vi "Andor_Cam.vi"(0 "Operation":T2(ring), 1 "Camera-specific in":variant, 5 "Exposure time (s)":dbl, 7 "Save path":path, 9 "Capture mode":enum16{"Single frame", "Sequence"}(ring), 11 "Capture button":refnum<vi>, 12 "Image in":variant, 14 "Frames in sequence":u32) -> (3 "Camera-specific out":variant, 4 "Status":T1)   [LabVIEW 2018]
uses:
  <userlib>/atmcd32d.llb/AcquisitionMode_mode typedef.ctl
  <userlib>/atmcd32d.llb/ReadMode_mode typedef.ctl
  <userlib>/atmcd32d.llb/HSSpeed_type typedef.ctl
  <userlib>/atmcd32d.llb/TriggerMode_mode typedef.ctl
  <userlib>/atmcd32d.llb/Shutter_type typedef.ctl
  <userlib>/atmcd32d.llb/Shutter_mode typedef.ctl
  <vilib>/vision/Image Controls.llb/IMAQ Image.ctl
  <userlib>/atmcd32d.llb/Error Code Enum typedef.ctl
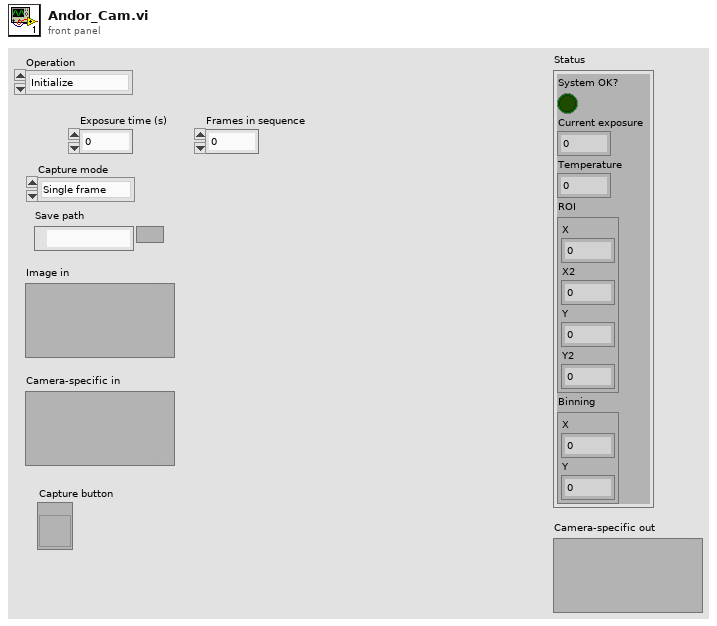
[diagram p1: front panel]
types:
  T1 = cluster{"System OK?":bool, "Current exposure":dbl, "Temperature":dbl, "ROI":cluster{"X":u32, "X2":u32, "Y":u32, "Y2":u32}, "Binning":cluster{"X":u32, "Y":u32}}
  T2 = enum16{"Initialize", "Shut down", "Set capture mode", "Set exposure", "Trigger and read", "Get status", "Other settings"}
  T3 = typedef "ReadMode_mode typedef.ctl" = enum16{"Full Vertical Binning", "Multi-Track", "Random-Track", "Single-Track", "Image"}
  T4 = typedef "HSSpeed_type typedef.ctl" = enum16{"EM Amp", "Conventional Amp"}
  T5 = typedef "TriggerMode_mode typedef.ctl" = enum16{"Internal", "External", "N/A (2)", "N/A (3)", "N/A (4)", "N/A (5)", "External Start", "External Exposure (Bulb)", "N/A (8)", "External FVB EM", "Software", "N/A (11)", "External Charge Shifting"}
  T6 = typedef "Shutter_mode typedef.ctl" = enum16{"Auto", "Open", "Close", "N/A (3)", "Open FVB Series", "Open Any Series"}
  T7 = typedef "AcquisitionMode_mode typedef.ctl" = enum16{"Reserved (0)", "Single Scan", "Accumulate", "Kinetics", "Fast Kinetics", "Run Till Abort", "Reserved (6)", "Reserved (7)", "Reserved (8)", "Time Delayed Integration"}
  T8 = typedef "IMAQ Image.ctl" = refnum<image>
  T9 = cluster{"New Image":T8, "Image":refnum<vi>, "FPS target":dbl}
  T10 = typedef "Error Code Enum typedef.ctl" = enum32{"N/A (0)", "DRV_ERROR_CODES", "DRV_SUCCESS", "DRV_VXDNOTINSTALLED", "DRV_ERROR_SCAN", "DRV_ERROR_CHECK_SUM", "DRV_ERROR_FILELOAD", "DRV_UNKNOWN_FUNC", "DRV_ERROR_VXD_INIT", "DRV_ERROR_ADDRESS", "DRV_ERROR_PAGELOCK", "DRV_ERROR_PAGEUNLOCK", "DRV_ERROR_BOARDTEST", "DRV_ERROR_ACK", "DRV_ERROR_UP_FIFO", "DRV_ERROR_PATTERN", "N/A (16)", "DRV_ACQUISITION_ERRORS", "DRV_ACQ_BUFFER", "DRV_ACQ_DOWNFIFO_FULL", "DRV_PROC_UNKONWN_INSTRUCTION", "DRV_ILLEGAL_OP_CODE", "DRV_KINETIC_TIME_NOT_MET", "DRV_ACCUM_TIME_NOT_MET", "DRV_NO_NEW_DATA", "N/A (25)", "DRV_SPOOLERROR", "N/A (27)", "N/A (28)", "N/A (29)", "N/A (30)", "N/A (31)", "N/A (32)", "DRV_TEMPERATURE_CODES", "DRV_TEMPERATURE_OFF", "DRV_TEMPERATURE_NOT_STABILIZED", "DRV_TEMPERATURE_STABILIZED", "DRV_TEMPERATURE_NOT_REACHED", "DRV_TEMPERATURE_OUT_RANGE", "DRV_TEMPERATURE_NOT_SUPPORTED", "DRV_TEMPERATURE_DRIFT", "N/A (41)", "N/A (42)", "N/A (43)", "N/A (44)", "N/A (45)", "N/A (46)", "N/A (47)", "N/A (48)", "DRV_GENERAL_ERRORS", "DRV_INVALID_AUX", "DRV_COF_NOTLOADED", "DRV_FPGAPROG", "DRV_FLEXERROR", "DRV_GPIBERROR", "N/A (55)", "N/A (56)", "N/A (57)", "N/A (58)", "N/A (59)", "N/A (60)", "N/A (61)", "N/A (62)", "N/A (63)", "DRV_DATATYPE", "DRV_DRIVER_ERRORS", "DRV_P1INVALID", "DRV_P2INVALID", "DRV_P3INVALID", "DRV_P4INVALID", "DRV_INIERROR", "DRV_COFERROR", "DRV_ACQUIRING", "DRV_IDLE", "DRV_TEMPCYCLE", "DRV_NOT_INITIALIZED", "DRV_P5INVALID", "DRV_P6INVALID", "DRV_INVALID_MODE", "DRV_INVALID_FILTER", "DRV_I2CERRORS", "DRV_I2CDEVNOTFOUND", "DRV_I2CTIMEOUT", "DRV_P7INVALID", "N/A (84)", "N/A (85)", "N/A (86)", "N/A (87)", "N/A (88)", "N/A (89)", "DRV_IOCERROR", "DRV_VRMVERSIONERROR"}
  T11 = enum16{"open", "replace", "create", "open or create", "replace or create", "replace or create with confirmation"}
  T12 = typedef "Shutter_type typedef.ctl" = enum16{"TTL Low", "TTL High"}
  T13 = cluster{"File refnum":refnum<file>, "Image File Directory":cluster{cluster{"Field":u16, "Type":u16, "Count":u32, "Value / Offset":u32, "Add IFD Offset?":bool}[], cluster{"Data":u32[], "Add offset?":bool}[]}, "Big endian?":bool, "IFD Offset Size":u32}
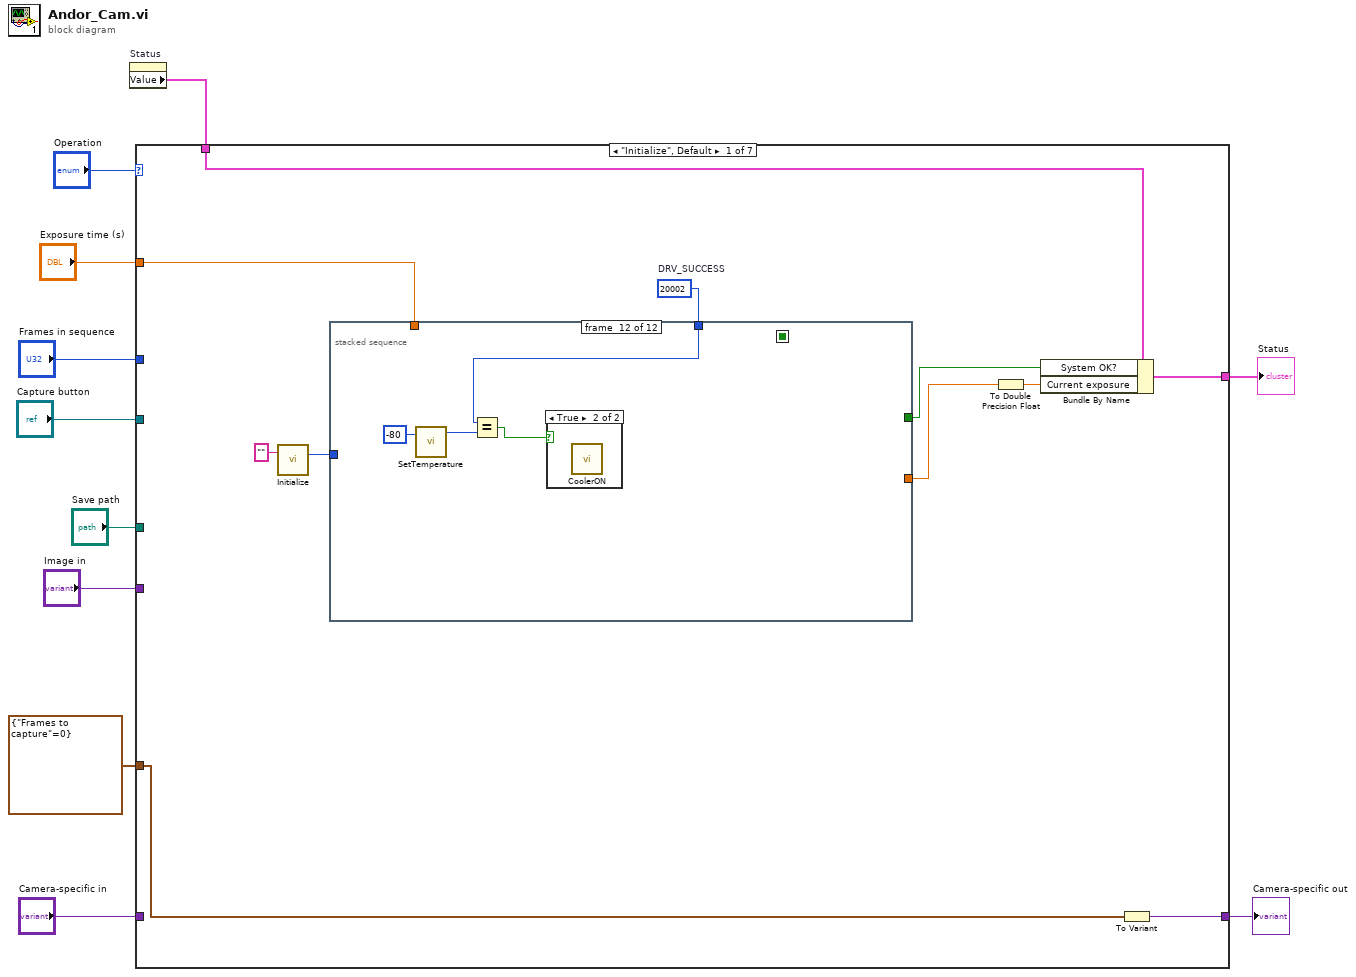
[diagram p0: block diagram]
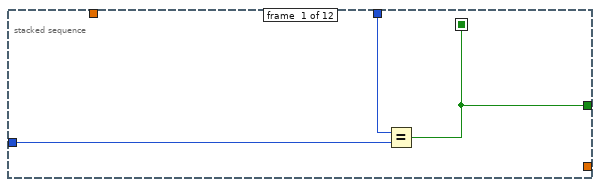
[diagram p2: hidden frame]
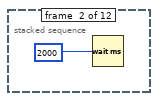
[diagram p3: hidden frame]
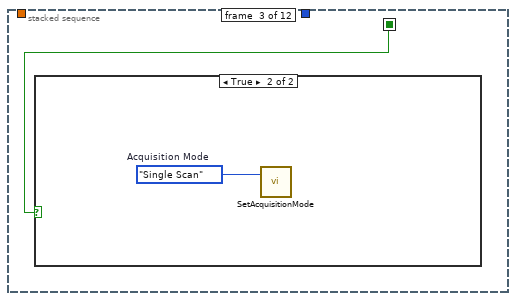
[diagram p4: hidden frame]
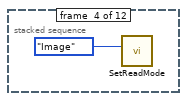
[diagram p6: hidden frame]
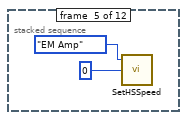
[diagram p7: hidden frame]
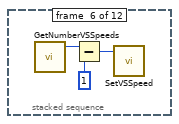
[diagram p8: hidden frame]
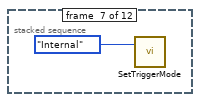
[diagram p9: hidden frame]
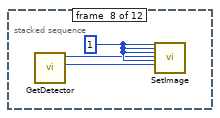
[diagram p10: hidden frame]
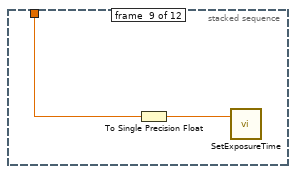
[diagram p11: hidden frame]
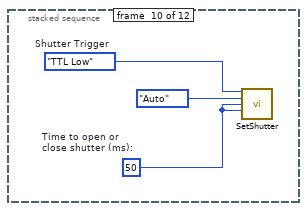
[diagram p12: hidden frame]
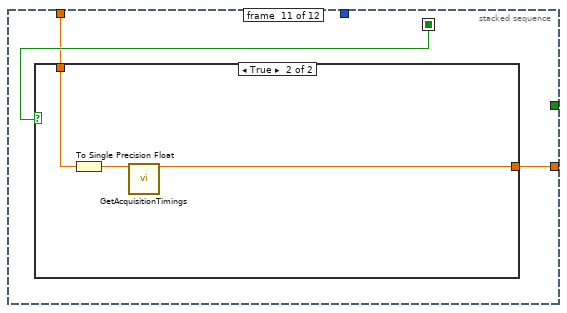
[diagram p13: hidden frame]
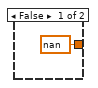
[diagram p14: hidden frame]
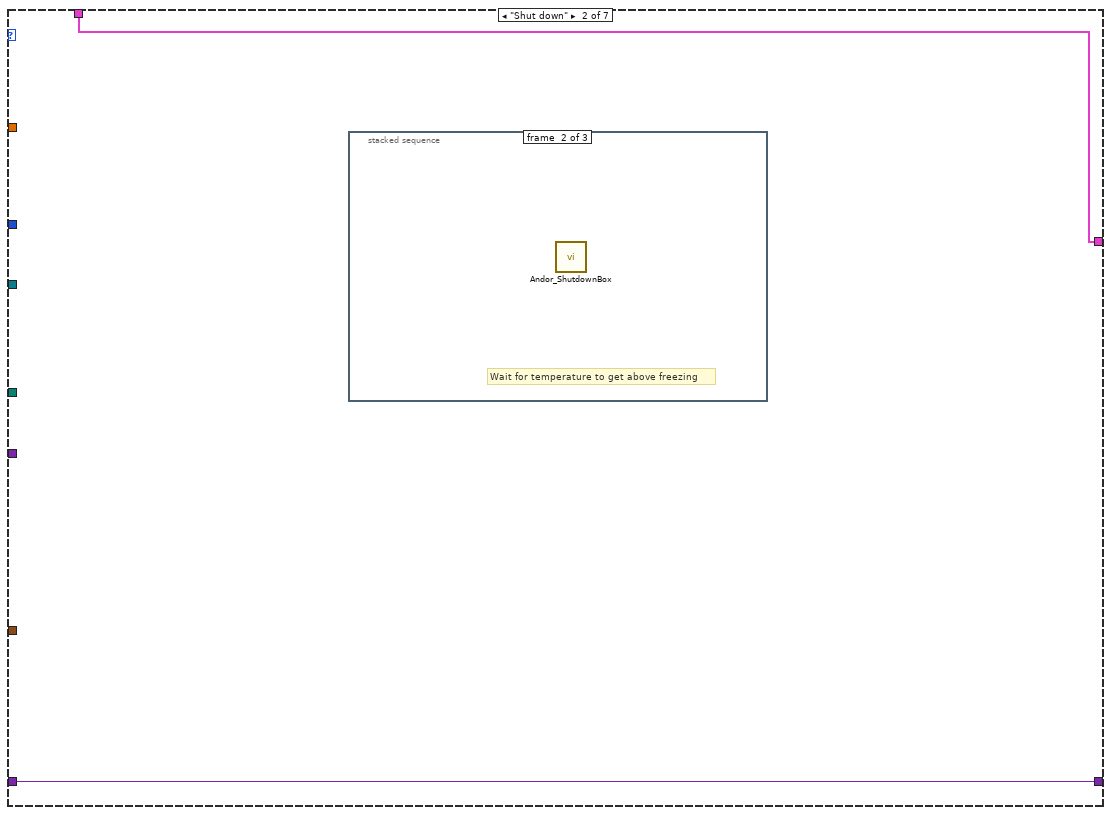
[diagram p16: hidden frame]
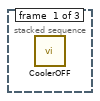
[diagram p17: hidden frame]
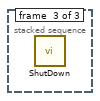
[diagram p18: hidden frame]
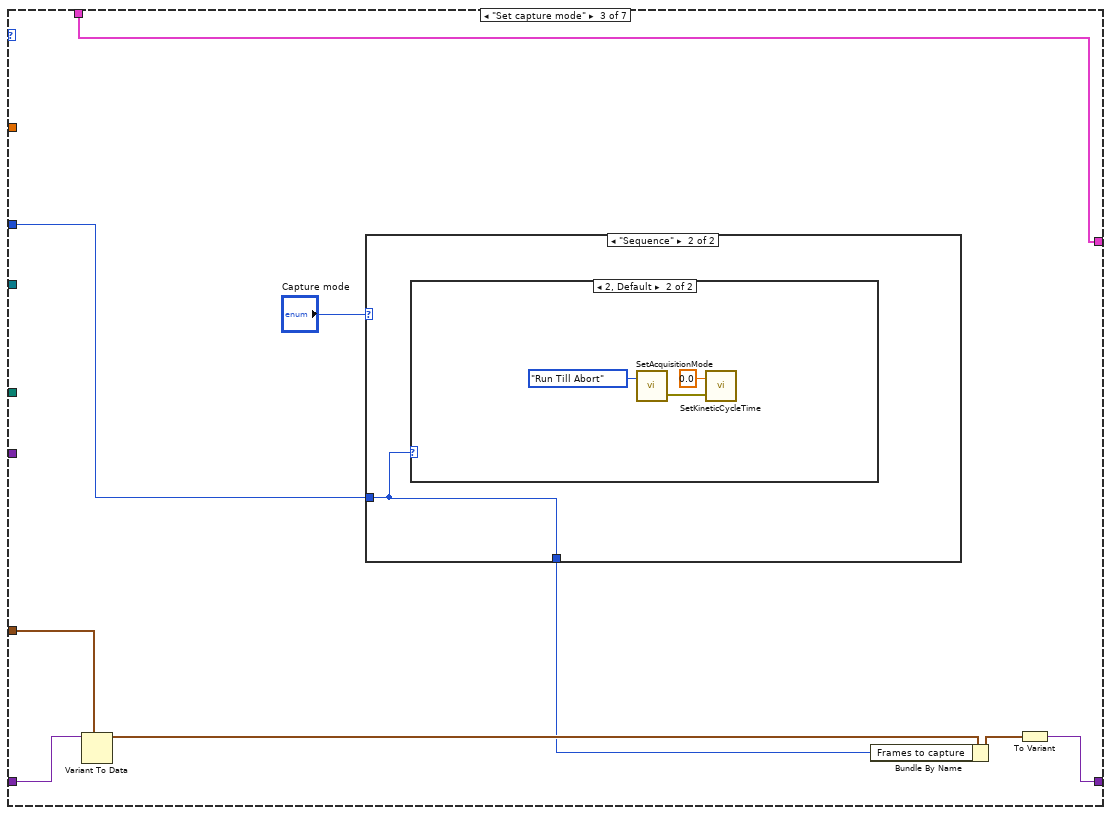
[diagram p19: hidden frame]
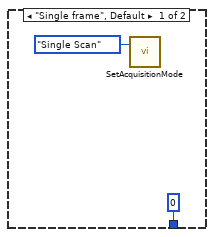
[diagram p20: hidden frame]
diagram:
  n1 = property on="Status" class="Clust (strict)"() -> ("Value"=w9:T1)  [unwired: 2 in, 2 out]
  n2 = case shown="\"Initialize\", Default" "Operation" {
    tunnel: "Exposure time (s)" -> [w19 _ _ w76 _ _ _]
    tunnel: w9 -> [w18 w56 w65 w78 w93 w321 w323]
    tunnel: [w17 w56 w65 w75 w93 w320 w323] -> w8
    tunnel: "Save path" -> [_ _ _ _ w92 _ _]
    tunnel: "Image in" -> [_ _ _ _ w85 _ _]
    tunnel: [w13 w55 w60 w73 w91 w316 w322] -> w5
    tunnel: "Camera-specific in" -> [_ w55 w63 w73 w91 w316 w322]
    tunnel: cluster{"Frames to capture":u32} {"Frames to capture"=0} -> [w14 _ w62 _ w90 _ _]
    tunnel: "Frames in sequence" -> [_ _ w57 _ _ _ _]
    tunnel: "Capture button" -> [_ _ _ _ w83 _ _]
    frame "Initialize", Default {
      w20 = u32 20002  # DRV_SUCCESS
      n3 = call <userlib>:"Initialize.vi"("directory (\"\")"="" ("directory (\"\")")) -> ("DLL error code"=w21:u32)  [unwired: 1 in, 1 out]
      n4 = stacked-sequence {
        seq-local: [w23 _ _ _ _ _ _ _ _ _ _ _] -> [_ _ w27 _ _ _ _ _ _ _ w46 _]
        tunnel: w19 -> [_ _ _ _ _ _ _ _ w40 _ w45 _]
        tunnel: w20 -> [w25 _ _ _ _ _ _ _ _ _ _ w52]
        tunnel: w21 -> [w24 _ _ _ _ _ _ _ _ _ _ _]
        tunnel: [w23 _ _ _ _ _ _ _ _ _ _ _] -> w16
        tunnel: [_ _ _ _ _ _ _ _ _ _ w44 _] -> w15
        frame #0 {
          n5 = Equal?(x=w25, y=w24) -> (x = y?=w23:bool)
        }
        frame #1 {
          n6 = Wait (ms)(milliseconds to wait=u32 2000) -> ()  [unwired: 1 out]
        }
        frame #2 {
          n7 = case shown="True" w27 {
            frame False {
            }
            frame True {
              w28 = AcquisitionMode_mode_typedef."Single Scan"  # Acquisition Mode
              n8 = call <userlib>:"SetAcquisitionMode.vi"("mode"=w28) -> ()  [unwired: 1 in, 2 out]
            }
          }
        }
        frame #3 {
          n9 = call <userlib>:"SetReadMode.vi"("mode"=ReadMode_mode_typedef."Image") -> ()  [unwired: 1 in, 2 out]
        }
        frame #4 {
          n10 = call <userlib>:"SetHSSpeed.vi"("index"=0, "type"=HSSpeed_type_typedef."EM Amp") -> ()  [unwired: 2 in, 2 out]
        }
        frame #5 {
          n11 = call <userlib>:"GetNumberVSSpeeds.vi"() -> ("number"=w34:i32)  [unwired: 3 in, 2 out]
          n12 = Subtract(x=w34, y=1) -> (x-y=w32:i32)
          n13 = call <userlib>:"SetVSSpeed.vi"("index"=w32) -> ()  [unwired: 1 in, 2 out]
        }
        frame #6 {
          n14 = call <userlib>:"SetTriggerMode.vi"("mode"=TriggerMode_mode_typedef."Internal") -> ()  [unwired: 1 in, 2 out]
        }
        frame #7 {
          w38 = 1 ("hbin")
          n15 = call <userlib>:"GetDetector.vi"() -> ("ypixels"=w36:i32, "xpixels"=w37:i32)  [unwired: 4 in, 2 out]
          n16 = call <userlib>:"SetImage.vi"("hbin"=w38, "vbin"=w38, "hstart"=w38, "hend"=w37, "vstart"=w38, "vend"=w36) -> ()  [unwired: 20 in, 2 out]
        }
        frame #8 {
          n17 = To Single Precision Float(number=w40) -> (single precision float=w39:sgl)
          n18 = call <userlib>:"SetExposureTime.vi"("time"=w39) -> ()  [unwired: 1 in, 2 out]
        }
        frame #9 {
          w43 = 50  # Time to open or close shutter (ms):
          w42 = Shutter_type_typedef."TTL Low"  # Shutter Trigger
          n19 = call <userlib>:"SetShutter.vi"("type"=w42, "mode"=Shutter_mode_typedef."Auto", "closingtime"=w43, "openingtime"=w43) -> ()  [unwired: 10 in, 2 out]
        }
        frame #10 {
          n20 = case shown="True" w46 {
            tunnel: w45 -> [_ w50]
            tunnel: [sgl nan ("exposure") w49] -> w44
            frame False {
            }
            frame True {
              n21 = To Single Precision Float(number=w50) -> (single precision float=w48:sgl)
              n22 = call <userlib>:"GetAcquisitionTimings.vi"("exposure input"=w48) -> ("exposure"=w49:sgl)  [unwired: 10 in, 4 out]
            }
          }
        }
        frame #11 {
          n23 = call <userlib>:"SetTemperature.vi"("temperature"=-80) -> ("DLL error code"=w53:u32)  [unwired: 1 in, 1 out]
          n24 = Equal?(x=w52, y=w53) -> (x = y?=w51:bool)
          n25 = case shown="True" w51 {
            frame False {
            }
            frame True {
              n26 = call <userlib>:"CoolerON.vi"() -> ()  [unwired: 2 in, 2 out]
            }
          }
        }
      }
      n27 = To Double Precision Float(number=w15) -> (double precision float=w12:dbl)
      n28 = Bundle By Name(cluster=w18, "System OK?"=w16, "Current exposure"=w12) -> (w17:T1)
      n29 = To Variant(anything=w14) -> (Variant=w13:variant)
    }
    frame "Shut down" {
      n30 = stacked-sequence {
        frame #0 {
          n31 = call <userlib>:"CoolerOFF.vi"() -> ()  [unwired: 2 in, 2 out]
        }
        frame #1 {
          # "Wait for temperature to get above freezing"
          n32 = call "Andor_ShutdownBox.vi"() -> ()  [unwired: 12 in]
        }
        frame #2 {
          n33 = call <userlib>:"ShutDown.vi"() -> ()  [unwired: 2 in, 2 out]
        }
      }
    }
    frame "Set capture mode" {
      n34 = Variant To Data(type=w62, Variant=w63) -> (data=w61:cluster{"Frames to capture":u32})  [unwired: 1 in, 1 out]
      n35 = case shown="\"Sequence\"" "Capture mode" {
        tunnel: [u32 0 ("Frames in sequence") w68] -> w58
        tunnel: w57 -> [_ w68]
        frame "Single frame", Default {
          n36 = call <userlib>:"SetAcquisitionMode.vi"("mode"=AcquisitionMode_mode_typedef."Single Scan") -> ()  [unwired: 1 in, 2 out]
        }
        frame "Sequence" {
          n37 = case shown="2, Default" w68 {
            frame 0, 1 {
              n38 = call <userlib>:"SetAcquisitionMode.vi"("mode"=AcquisitionMode_mode_typedef."Single Scan") -> ()  [unwired: 1 in, 2 out]
            }
            frame 2, Default {
              n39 = call <userlib>:"SetAcquisitionMode.vi"("mode"=AcquisitionMode_mode_typedef."Run Till Abort") -> ("error out"=w70:errorcluster)  [unwired: 1 in, 1 out]
              n40 = call <userlib>:"SetKineticCycleTime.vi"("error in (no error)"=w70, "time"=sgl 0.0) -> ()  [unwired: 2 out]
            }
          }
        }
      }
      n41 = Bundle By Name(cluster=w61, "Frames to capture"=w58) -> (w59:cluster{"Frames to capture":u32})
      n42 = To Variant(anything=w59) -> (Variant=w60:variant)
    }
    frame "Set exposure" {
      n43 = To Single Precision Float(number=w76) -> (single precision float=w77:sgl)
      n44 = stacked-sequence {
        tunnel: w77 -> [w79 w81]
        tunnel: [_ w80] -> w74
        frame #0 {
          n45 = call <userlib>:"SetExposureTime.vi"("time"=w79) -> ()  [unwired: 1 in, 2 out]
        }
        frame #1 {
          n46 = call <userlib>:"GetAcquisitionTimings.vi"("exposure input"=w81) -> ("exposure"=w80:sgl)  [unwired: 10 in, 4 out]
        }
      }
      n47 = Bundle By Name(cluster=w78, "Current exposure"=w74) -> (w75:T1)
    }
    frame "Trigger and read" {
      n48 = Variant To Data(type=w90, Variant=w91) -> (data=w89:cluster{"Frames to capture":u32})  [unwired: 1 in, 1 out]
      n49 = Unbundle By Name(w89) -> ("Frames to capture"=w88:u32)
      n50 = Variant To Data(type=T9 {"New Image"=refnum, "Image"=refnum, "FPS target"=0.0} ("output cluster"), Variant=w85) -> (data=w87:T9)  [unwired: 1 in, 1 out]
      n51 = Unbundle(w87) -> ("New Image"=w84:T8, "Image"=w82:refnum<vi>)  [unwired: 1 out]
      n52 = case shown="2, Default" w88 {
        selector: w88 -> [_ w151]
        tunnel: w92 -> [w96 w154]
        tunnel: w84 -> [w95 w153]
        tunnel: w83 -> [_ w152]
        tunnel: w82 -> [w94 w150]
        frame 0, 1 {
          n53 = stacked-sequence {
            seq-local: [w99 _ _] -> [_ w100 _]
            tunnel: w96 -> [_ _ w112]
            tunnel: w95 -> [_ _ w110]
            tunnel: w94 -> [_ _ w105]
            frame #0 {
              w97 = u32 20002  # DRV_SUCCESS
              n54 = call <userlib>:"StartAcquisition.vi"() -> ("DLL error code"=w98:u32)  [unwired: 2 in, 1 out]
              n55 = Equal?(x=w97, y=w98) -> (x = y?=w99:bool)
            }
            frame #1 {
              n56 = case shown="True" w100 {
                frame False {
                }
                frame True {
                  n57 = while {
                    stop <- w103 continue-if-true
                    n58 = call <userlib>:"GetStatus.vi"() -> ("status"=w102:T10)  [unwired: 3 in, 2 out]
                    n59 = Wait Until Next ms Multiple(millisecond multiple=u32 25) -> ()  [unwired: 1 out]
                    n60 = Equal?(x=w102, y=Error_Code_Enum_typedef."DRV_ACQUIRING" ("status")) -> (x = y?=w103:bool)
                  }
                }
              }
            }
            frame #2 {
              n61 = call <userlib>:"GetDetector.vi"() -> ("ypixels"=w106:i32, "xpixels"=w107:i32)  [unwired: 4 in, 2 out]
              n62 = Multiply(x=w107, y=w106) -> (x*y=w118:i32)
              n63 = To Unsigned Long Integer(number=w118) -> (unsigned 32bit integer=w114:u32)
              n64 = Not A Number/Path/Refnum?(number/path/refnum=w110) -> (NaN/Path/Refnum?=w109:bool)
              n65 = call <userlib>:"GetAcquiredData.vi"("size"=w114) -> ("array"=w116:i32[])  [unwired: 2 in, 2 out]
              n66 = Multiply(x=1, y=w116) -> (x*y=w115:i32[])
              n67 = Reshape Array(w115, w106, w107) -> (w111:i32[][])
              n68 = To Unsigned Word Integer(number=w111) -> (unsigned 16bit integer=w108:u16[][])
              n69 = case shown="False" w109 {
                tunnel: w110 -> [w122 _]
                tunnel: w108 -> [w121 _]
                tunnel: w105 -> [w120 _]
                frame False {
                  n70 = call "IMAQ ArrayToImage"("Image Pixels (U16)"=w121, "Image"=w122) -> ("Image Out"=w119:T8)  [unwired: 8 in, 1 out]
                  n71 = property class="ImageControl"(reference=w120, "Value"=w119) -> ()  [unwired: 1 in, 2 out]
                }
                frame True {
                }
              }
              n72 = Not A Number/Path/Refnum?(number/path/refnum=w112) -> (NaN/Path/Refnum?=w113:bool)
              n73 = case shown="False" w113 {
                tunnel: w112 -> [w126 _]
                tunnel: w108 -> [w127 _]
                tunnel: w107 -> [w124 _]
                tunnel: w106 -> [w123 _]
                frame False {
                  n74 = call <vilib>:"Get File Extension.vi"("file"=w126) -> ("lowercase file extension"=w125:string)  [unwired: 6 in, 4 out]
                  n75 = case shown="\"'tiff'\", \"tif\"" w125 {
                    tunnel: w126 -> [w142 w149]
                    tunnel: w127 -> [w132 w147]
                    tunnel: w124 -> [w140 _]
                    tunnel: w123 -> [w139 _]
                    frame "'tiff'", "tif" {
                      n76 = To Unsigned Long Integer(number=w139) -> (unsigned 32bit integer=w128:u32)
                      n77 = To Unsigned Long Integer(number=w140) -> (unsigned 32bit integer=w129:u32)
                      n78 = call "TIFFStream Open.vi"("Bytes per strip"=u32 8000, "File path"=w142, "Height Pixels"=w128, "Width Pixels"=w129, "Big endian?"=FALSE) -> ("error out"=w136:errorcluster, "Current and next IFD offset"=w134:u32[], "Image data reference"=w133:refnum<data-value>, "File data"=w138:T13)  [unwired: 3 in]
                      n79 = in-place {
                        in-place-border: w132 -> [w143]
                        n80 = in-place-dvr #1(w133) -> ()  [unwired: 2 out]
                        n81 = in-place-dvr #1(w143) -> (w131:refnum<data-value>)  [unwired: 1 out]
                      }
                      n82 = call "TIFFStream Write.vi"("File data"=w138, "error in (no error)"=w136, "Last image in file?"=TRUE, "Current and next IFD offset in"=w134, "Image data reference"=w131) -> ("error out"=w137:errorcluster)  [unwired: 4 in, 2 out]
                      n83 = call "TIFFStream Close.vi"("error in (no error)"=w137, "Image data reference"=w131, "File data"=w138) -> ()  [unwired: 8 in, 1 out]
                    }
                    frame "dat", Default {
                      n84 = Open/Create/Replace File(file path (use dialog)=w149, operation (0:open)=T11."replace or create") -> (refnum out=w148:refnum<file>)  [unwired: 4 in, 2 out]
                      n85 = Write to Binary File(file (use dialog)=w148, data=w147, 5:FALSE ("prepend array or string size? (T)")) -> (refnum out=w145:refnum<file>)  [unwired: 3 in, 2 out]
                      n86 = Close File(refnum=w145) -> ()  [unwired: 1 in, 2 out]
                    }
                  }
                }
                frame True {
                }
              }
            }
          }
        }
        frame 2, Default {
          n87 = stacked-sequence {
            seq-local: [_ w193 _ _ _] -> [_ _ _ _ _]
            seq-local: [w158 _ _ _ _] -> [_ _ w205 _ _]
            seq-local: [w166 _ _ _ _] -> [_ _ w207 _ w303]
            seq-local: [w162 _ _ _ _] -> [_ _ w204 _ _]
            seq-local: [w163 _ _ _ _] -> [_ _ w206 _ _]
            seq-local: [w161 _ _ _ _] -> [_ _ w203 _ _]
            seq-local: [w160 _ _ _ _] -> [_ _ w201 _ w300]
            seq-local: [w159 _ _ _ _] -> [_ _ w202 _ _]
            seq-local: [_ _ w200 _ _] -> [_ _ _ _ w299]
            seq-local: [_ _ w199 _ _] -> [_ _ _ _ w298]
            seq-local: [w156 _ _ _ _] -> [_ _ w198 _ _]
            seq-local: [w155 _ _ _ _] -> [_ _ w197 _ _]
            tunnel: w154 -> [w168 _ w210 _ w301]
            tunnel: w153 -> [_ _ w209 _ _]
            tunnel: w152 -> [_ _ w208 _ _]
            tunnel: w151 -> [_ _ w196 _ _]
            tunnel: w150 -> [_ _ w194 _ _]
            frame #0 {
              n88 = call <userlib>:"GetDetector.vi"() -> ("ypixels"=w162:i32, "xpixels"=w163:i32)  [unwired: 4 in, 2 out]
              n89 = To Unsigned Long Integer(number=w163) -> (unsigned 32bit integer=w165:u32)
              n90 = To Unsigned Long Integer(number=w162) -> (unsigned 32bit integer=w164:u32)
              n91 = Multiply(x=w165, y=w164) -> (x*y=w158:u32)
              n92 = Not A Number/Path/Refnum?(number/path/refnum=w168) -> (NaN/Path/Refnum?=w167:bool)
              n93 = Initialize Array(0 ("element"), w158) -> (w156:i32[])
              n94 = case shown="False" w167 {
                tunnel: w168 -> [w177 _]
                tunnel: w165 -> [w175 _]
                tunnel: w164 -> [w174 _]
                tunnel: [w173 _] -> w166
                tunnel: [w172 _] -> w161
                tunnel: [w171 _] -> w160
                tunnel: [w170 _] -> w159
                tunnel: [w169 _] -> w155
                frame False {
                  n95 = call <vilib>:"Get File Extension.vi"("file"=w177) -> ("lowercase file extension"=w176:string)  [unwired: 6 in, 4 out]
                  n96 = case shown="\"dat\", Default" w176 {
                    tunnel: w177 -> [w186 w190]
                    tunnel: w175 -> [w182 _]
                    tunnel: w174 -> [w183 _]
                    tunnel: [_ w188] -> w173
                    tunnel: [w181 _] -> w172
                    tunnel: [w180 _] -> w171
                    tunnel: [w179 _] -> w170
                    tunnel: [w178 w187] -> w169
                    frame "'tiff'", "tif" {
                      n97 = call "TIFFStream Open.vi"("Bytes per strip"=u32 8000, "File path"=w186, "Height Pixels"=w183, "Width Pixels"=w182, "Big endian?"=FALSE) -> ("error out"=w178:errorcluster, "Current and next IFD offset"=w179:u32[], "Image data reference"=w180:refnum<data-value>, "File data"=w181:T13)  [unwired: 3 in]
                    }
                    frame "dat", Default {
                      n98 = Open/Create/Replace File(file path (use dialog)=w190, operation (0:open)=T11."replace or create") -> (refnum out=w188:refnum<file>, error out=w187:errorcluster)  [unwired: 4 in, 1 out]
                    }
                  }
                }
                frame True {
                }
              }
            }
            frame #1 {
              w191 = u32 20002  # DRV_SUCCESS
              n99 = call <userlib>:"StartAcquisition.vi"() -> ("DLL error code"=w192:u32)  [unwired: 2 in, 1 out]
              n100 = Equal?(x=w191, y=w192) -> (x = y?=w193:bool)
            }
            frame #2 {
              n101 = while {
                tunnel: w210 -> [w239]
                tunnel: w209 -> [w238]
                tunnel: w208 -> [w223]
                tunnel: w207 -> [w234]
                tunnel: w206 -> [w222]
                tunnel: w205 -> [w233]
                tunnel: w204 -> [w232]
                shift-right: [w231] -> w199
                shift-left: w202 -> [w230]
                shift-right: [w229] -> w200
                shift-left: w203 -> [w228]
                shift-right: [w227] -> _
                shift-left: w197 -> [w225]
                tunnel: w201 -> [w226]
                tunnel: w198 -> [w224]
                tunnel: w196 -> [w219]
                border: u32 0 -> [_]
                tunnel: w194 -> [w211]
                stop <- w215 continue-if-true
                n102 = call <userlib>:"GetOldestImage.vi"("size"=w233, "array"=w224) -> ("array"=w237:i32[], "DLL error code"=w221:u32)  [unwired: 1 in, 1 out]
                n103 = property class="Bool (strict)"(reference=w223) -> ("Value"=w216:bool)  [unwired: 1 in, 2 out]
                n104 = Equal?(x=w221, y=u32 20002) -> (x = y?=w220:bool)
                n105 = feedback #2() -> (w213:u32)
                n106 = case shown="True" w220 {
                  tunnel: w239 -> [_ w262]
                  tunnel: w238 -> [_ w260]
                  tunnel: w237 -> [_ w258]
                  tunnel: w234 -> [_ w257]
                  tunnel: w232 -> [_ w256]
                  tunnel: [w242 w255] -> w231
                  tunnel: w230 -> [w242 w254]
                  tunnel: [w243 w253] -> w229
                  tunnel: w228 -> [w243 w252]
                  tunnel: [w241 w251] -> w227
                  tunnel: w226 -> [_ w250]
                  tunnel: w225 -> [w241 w249]
                  tunnel: w222 -> [_ w247]
                  tunnel: [w240 w246] -> w212
                  tunnel: w213 -> [w240 w245]
                  tunnel: w211 -> [_ w244]
                  frame False {
                  }
                  frame True {
                    n107 = Not A Number/Path/Refnum?(number/path/refnum=w260) -> (NaN/Path/Refnum?=w259:bool)
                    n108 = Multiply(x=1, y=w258) -> (x*y=w264:i32[])
                    n109 = Reshape Array(w264, w256, w247) -> (w261:i32[][])
                    n110 = To Unsigned Word Integer(number=w261) -> (unsigned 16bit integer=w248:u16[][])
                    n111 = case shown="False" w259 {
                      tunnel: w260 -> [w269 _]
                      tunnel: w248 -> [w268 _]
                      tunnel: w244 -> [w267 _]
                      frame False {
                        n112 = call "IMAQ ArrayToImage"("Image Pixels (U16)"=w268, "Image"=w269) -> ("Image Out"=w266:T8)  [unwired: 8 in, 1 out]
                        n113 = property class="ImageControl"(reference=w267, "Value"=w266) -> ()  [unwired: 1 in, 2 out]
                      }
                      frame True {
                      }
                    }
                    n114 = Not A Number/Path/Refnum?(number/path/refnum=w262) -> (NaN/Path/Refnum?=w263:bool)
                    n115 = case shown="False" w263 {
                      tunnel: w262 -> [w279 _]
                      tunnel: w248 -> [w280 _]
                      tunnel: w257 -> [w277 _]
                      tunnel: [w276 _] -> w255
                      tunnel: w254 -> [w275 _]
                      tunnel: [w274 _] -> w253
                      tunnel: w252 -> [w273 _]
                      tunnel: [w272 w297] -> w251
                      tunnel: w250 -> [w271 _]
                      tunnel: w249 -> [w270 w297]
                      frame False {
                        n116 = call <vilib>:"Get File Extension.vi"("file"=w279) -> ("lowercase file extension"=w278:string)  [unwired: 6 in, 4 out]
                        n117 = case shown="\"'tiff'\", \"tif\"" w278 {
                          tunnel: w280 -> [w289 w296]
                          tunnel: w277 -> [_ w294]
                          tunnel: [w287 _] -> w276
                          tunnel: w275 -> [w286 _]
                          tunnel: [w285 _] -> w274
                          tunnel: w273 -> [w284 _]
                          tunnel: [w283 w293] -> w272
                          tunnel: w271 -> [w282 _]
                          tunnel: w270 -> [w281 w292]
                          frame "'tiff'", "tif" {
                            n118 = in-place {
                              in-place-border: w289 -> [w291]
                              n119 = in-place-dvr #3(w282) -> ()  [unwired: 2 out]
                              n120 = in-place-dvr #3(w291) -> (w288:refnum<data-value>)  [unwired: 1 out]
                            }
                            n121 = call "TIFFStream Write.vi"("File data"=w284, "error in (no error)"=w281, "Last image in file?"=TRUE, "Current and next IFD offset in"=w286, "Image data reference"=w288) -> ("error out"=w283:errorcluster, "Current and next IFD offset out"=w287:u32[], "File data out"=w285:T13)  [unwired: 4 in]
                          }
                          frame "dat", Default {
                            n122 = Write to Binary File(file (use dialog)=w294, data=w296, error in=w292, 5:FALSE ("prepend array or string size? (T)")) -> (error out=w293:errorcluster)  [unwired: 2 in, 2 out]
                          }
                        }
                      }
                      frame True {
                      }
                    }
                    n123 = Increment(x=w245) -> (x+1=w246:u32)
                  }
                }
                n124 = feedback-in #2(w212) -> ()
                n125 = Less?(x=w212, y=w219) -> (x < y?=w218:bool)
                n126 = call <userlib>:"GetStatus.vi"() -> ("status"=w236:T10)  [unwired: 3 in, 2 out]
                n127 = Equal?(x=w236, y=Error_Code_Enum_typedef."DRV_ACQUIRING" ("status")) -> (x = y?=w217:bool)
                n128 = Compound Arithmetic op=AND(w216, w217, w218) -> (w215:bool)
              }
            }
            frame #3 {
              # "Stop capture"
              n129 = call <userlib>:"AbortAcquisition.vi"() -> ()  [unwired: 2 in, 2 out]
            }
            frame #4 {
              n130 = Not A Number/Path/Refnum?(number/path/refnum=w301) -> (NaN/Path/Refnum?=w302:bool)
              n131 = case shown="False" w302 {
                tunnel: w301 -> [w309 _]
                tunnel: w303 -> [w307 _]
                tunnel: w300 -> [w306 _]
                tunnel: w299 -> [w305 _]
                tunnel: w298 -> [w304 _]
                frame False {
                  n132 = call <vilib>:"Get File Extension.vi"("file"=w309) -> ("lowercase file extension"=w308:string)  [unwired: 6 in, 4 out]
                  n133 = case shown="\"'tiff'\", \"tif\"" w308 {
                    tunnel: w307 -> [_ w313]
                    tunnel: w306 -> [w312 _]
                    tunnel: w305 -> [w311 _]
                    tunnel: w304 -> [w310 _]
                    frame "'tiff'", "tif" {
                      n134 = call "TIFFStream Close.vi"("Current and next IFD offset"=w310, "Image data reference"=w312, "File data"=w311) -> ()  [unwired: 8 in, 1 out]
                    }
                    frame "dat", Default {
                      n135 = Close File(refnum=w313) -> ()  [unwired: 1 in, 2 out]
                    }
                  }
                }
                frame True {
                }
              }
            }
          }
        }
      }
    }
    frame "Get status" {
      n136 = call <userlib>:"GetTemperature.vi"() -> ("status"=w318:T10, "temperature"=w319:i32)  [unwired: 4 in, 2 out]
      n137 = Equal?(x=Error_Code_Enum_typedef."DRV_SUCCESS", y=w318) -> (x = y?=w317:bool)
      n138 = To Double Precision Float(number=w319) -> (double precision float=w314:dbl)
      n139 = Bundle By Name(cluster=w321, "System OK?"=w317, "Temperature"=w314) -> (w320:T1)
    }
    frame "Other settings" {
      n140 = call "Andor_Settings.vi"() -> ()  [unwired: 12 in]
    }
  }
  "Status" <- w8
  "Camera-specific out" <- w5
